vi "autospotglobal.vi"(6 "Image In":T1, 7 "Enum":T2(ring)) -> (2 "New Image":T1)   [LabVIEW 2009]
uses:
  <vilib>/vision/Image Controls.llb/IMAQ Image.ctl
  <vilib>/vision/NI_Vision_Development_Module.lvlib
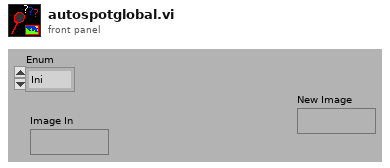
[diagram p1: front panel]
types:
  T1 = typedef "IMAQ Image.ctl" = refnum<image>
  T2 = enum16{"Ini", "get", "dump", "set", "draw", "black"}
  T3 = enum32{"Gray", "Binary", "Gradient", "Rainbow", "Temperature"}
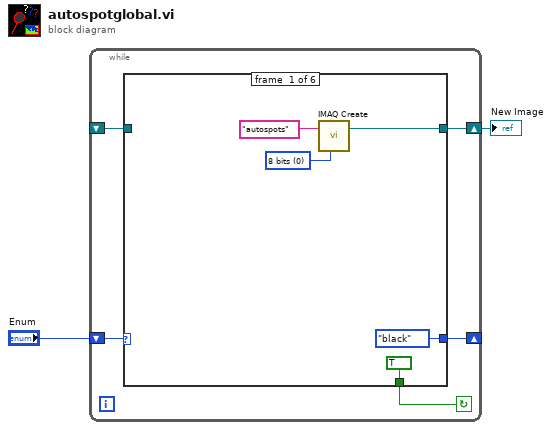
[diagram p0: block diagram]
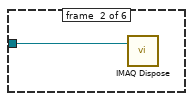
[diagram p2: hidden frame]
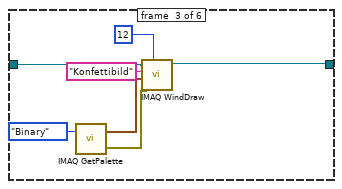
[diagram p3: hidden frame]
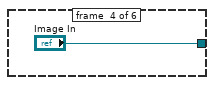
[diagram p4: hidden frame]
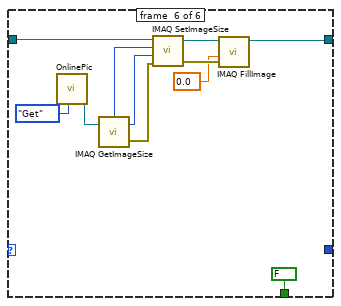
[diagram p6: hidden frame]
diagram:
  n1 = while {
    shift-right: [w7] -> w2
    shift-left: _ -> [w5]
    shift-right: [w3] -> _
    shift-left: "Enum" -> [w4]
    stop <- w6 continue-if-true
    n2 = case shown="\"set\"" w4 {
      tunnel: [w12 _ w19 "Image In" w22 w24] -> w7
      tunnel: [TRUE _ _ _ _ FALSE] -> w6
      tunnel: w5 -> [_ w13 w20 _ w22 w28]
      tunnel: [T2."black" ("Enum") _ _ _ _ _] -> w3
      frame #0 {
        w10 = u32 0 items=["8 bits", "16 bits", "Float", "Complex", "RGB", "HSL"] ("Image Type")
        n3 = call "IMAQ Create"("Image Name"="autospots", "Image Type"=w10) -> ("New Image"=w12:T1)  [unwired: 3 in, 1 out]
      }
      frame #1 {
        n4 = call "IMAQ Dispose"("Image"=w13) -> ()  [unwired: 5 in, 1 out]
      }
      frame #2 {
        n5 = call "IMAQ GetPalette"("Palette Number (gray)"=T3."Binary") -> ("Color Palette"=w16:cluster{"Red":u8, "Green":u8, "Blue":u8}[], "error out"=w14:errorcluster)  [unwired: 4 in]
        n6 = call "IMAQ WindDraw"("Window Number (0...15)"=12, "error in (no error)"=w14, "Color Palette"=w16, "Title"="Konfettibild", "Image"=w20) -> ("Image Out (duplicate)"=w19:T1)  [unwired: 5 in, 1 out]
      }
      frame #3 {
      }
      frame #4 {
      }
      frame #5 {
        n7 = call "OnlinePic.vi"("action"=enum16{"Get", "Set", "Change", "ini"}."Get" ("Enum")) -> ("Image Out (duplicate)"=w32:T1)  [unwired: 6 in, 4 out]
        n8 = call "IMAQ GetImageSize"("Image"=w32) -> ("Y Resolution"=w30:i32, "X Resolution"=w31:i32, "error out"=w29:errorcluster)  [unwired: 3 in]
        n9 = call "IMAQ SetImageSize"("error in (no error)"=w29, "Y Resolution"=w30, "X Resolution"=w31, "Image"=w28) -> ("error out"=w26:errorcluster, "Image Out"=w27:T1)  [unwired: 1 in]
        n10 = call "IMAQ FillImage"("error in (no error)"=w26, "Pixel Value (U8, U16, I16, Float)"=sgl 0.0 ("Pixel Value (U8, I16, Float)"), "Image"=w27) -> ("Image Out"=w24:T1)  [unwired: 7 in, 1 out]
      }
    }
  }
  "New Image" <- w2
